vi "Open and Configure Device 4RX.vi"(0 "USRP RIO Device":T14, 5 "reference frequency source":string(combo)="Internal", 9 "Wait for GPS Lock?":bool, 11 "error in":errorcluster, 12 "rx config":T2) -> (2 "rx channels":T4={"rx config"={"channel configuration"=[], "transfer mode"=enum."Finite", "sample rate"=10000000.0, "number of samples"=8192, "start trigger"=enum."Immediate"}, "reference frequency source"="Internal", "rx.data sink"=enum."Host", "rx.enabled channels"=[], "vertical range"=[], "rx.coerced configurations"={"coerced frequencies"=[], "coerced lo frequencies"=[], "coerced levels"=[], "coerced sample rates"=[]}} {"rx.coerced configurations"."coerced sample rates" format="%#.3pS/s"; "rx.coerced configurations"."coerced levels" format="%#.3gdBm"; "rx.coerced configurations"."coerced lo frequencies" format="%#.3pHz"; "rx.coerced configurations"."coerced frequencies" format="%#.3pHz"; "rx config"."channel configuration"."channel configuration"."frequency" format="%#.3pHz"; "rx config"."channel configuration"."channel configuration"."lo frequency" format="%#.3pHz"; "rx config"."channel configuration"."channel configuration"."level" format="%#_gdBm"; "rx config"."sample rate" format="%#.3pS/s"; "vertical range" format="%#.3pVpp"}, 4 "niUsrpRio Session (out)":T5 {"Daughterboard Clock Rate" format="%#.3pHz"; "FPGA Data Clock Rate" format="%#.3pHz"; "Data Clock Rate" format="%#.3pHz"; "Characterization Data"."Frequencies [Hz]" format="%#_6p"; "EEPROM Characterization Header"."Pointer to Device Data Header" format="%x"; "EEPROM Characterization Header"."Checksum" format="%x"; "Device Data Header"."Pointer to Characterization Data" format="%x"; "Device Data Header"."Checksum" format="%x"; "EEPROM Header"."Pointer to User Header" format="%x"; "EEPROM Header"."Pointer to Factory Header" format="%x"; "EEPROM Header"."Product Code" format="%x"; "EEPROM Header"."Checksum" format="%x"}, 6 "rx.coerced configurations":T3 caption="Rx" {"coerced if2 frequencies" format="%#.3pHz"; "coerced sample rates" format="%#.3pS/s"; "coerced gain" format="%#.2f"; "coerced if1 frequencies" format="%#.3pHz"; "coerced frequencies" format="%#.3pHz"}, 15 "error out":errorcluster)   [LabVIEW 2021]
uses:
  <vilib>/userdefined/Silver/nirio_resource_slv.ctl
  <instrlib>/niUsrpRio/Config/v1/Host/Public/niUsrpRio Session.ctl
  <instrlib>/_niInstr/Register Bus/v0/Host/Public/Register Bus Session.ctl
  <instrlib>/_niInstr/Register Bus/v0/Host/Private/Session Data.ctl
  <instrlib>/niUsrpRio/Config/v1/Host/Private/DB Queue Reference.ctl
  <instrlib>/niUsrpRio/Config/v1/Host/Private/Daughterboard Data.ctl
  <instrlib>/niUsrpRio/Config/v1/Host/Private/ATR state data.ctl
  <instrlib>/niUsrpRio/Config/v1/Host/Private/Antenna Configuration.ctl
  <instrlib>/niUsrpRio/Config/v1/Host/Private/CPLD Power Mode.ctl
  <instrlib>/niUsrpRio/Config/v1/Host/Public/EEPROM Header.ctl
  <instrlib>/niUsrpRio/Config/v1/Host/Public/EEPROM Device Data Header.ctl
  <instrlib>/niUsrpRio/Config/v1/Host/Public/EEPROM Characterization Header.ctl
  <instrlib>/niUsrpRio/Config/v1/Host/Public/Characterization Data.ctl
  <instrlib>/niUsrpRio/Config/v1/Host/Public/IQ Imbalance.ctl
  Rx Channels.ctl
  Start Trigger.ctl
  <instrlib>/_niInstr/Register Bus/v0/Host/niInstr Register Bus v0 Host.lvlib
  <instrlib>/niUsrpRio/Config/v1/Host/niUsrpRio Config v1 Host.lvlib
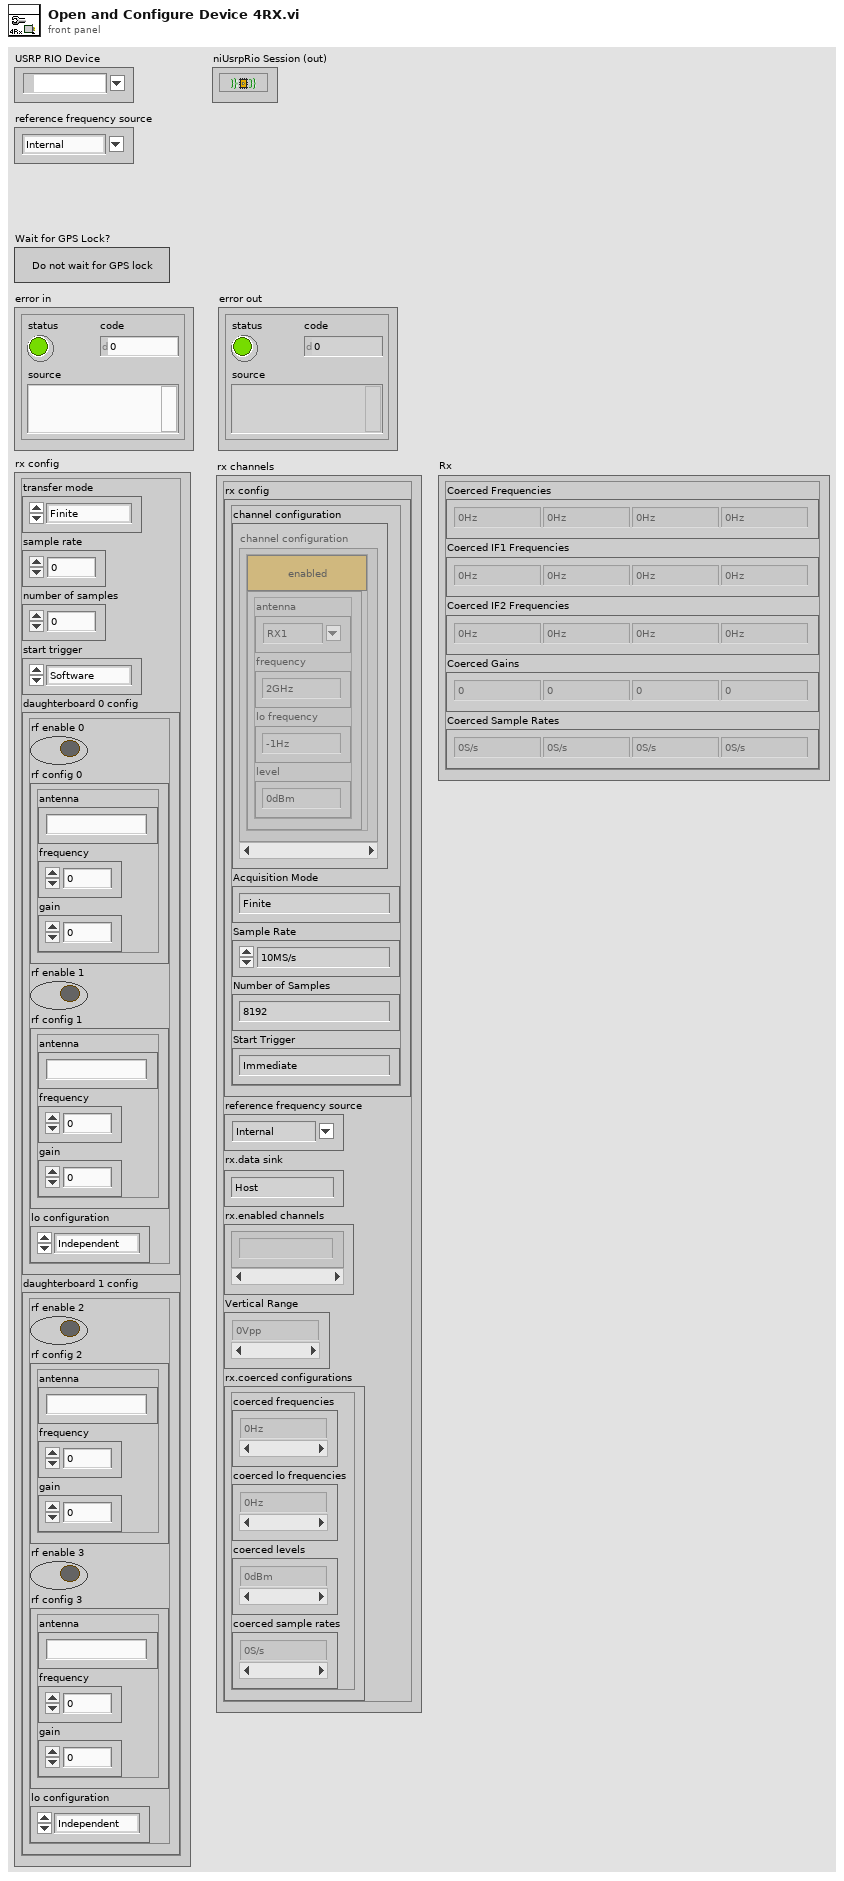
[diagram p1: front panel]
types:
  T1 = typedef "Start Trigger.ctl" = enum8{"Software", "Digital Edge", "Rx Start Trigger", "Tx Start Trigger", "Immediate", "Future Time Event"}
  T2 = cluster{"transfer mode":enum16{"Finite", "Continuous"}, "sample rate":dbl, "number of samples":u32, "start trigger":T1, "daughterboard 0 config":cluster{"rf enable 0":bool, "rf config 0":cluster{"antenna":string, "frequency":dbl, "gain":dbl}, "rf enable 1":bool, "rf config 1":cluster{"antenna":string, "frequency":dbl, "gain":dbl}, "lo configuration":enum16{"Independent", "Import", "Shared and Export", "Reimport", "Shared"}}, "daughterboard 1 config":cluster{"rf enable 2":bool, "rf config 2":cluster{"antenna":string, "frequency":dbl, "gain":dbl}, "rf enable 3":bool, "rf config 3":cluster{"antenna":string, "frequency":dbl, "gain":dbl}, "lo configuration":enum16{"Independent", "Import", "Shared and Export", "Reimport", "Shared"}}}
  T3 = cluster{"coerced frequencies":dbl[], "coerced if1 frequencies":dbl[], "coerced if2 frequencies":dbl[], "coerced gain":dbl[], "coerced sample rates":dbl[]}
  T4 = typedef "Rx Channels.ctl" = cluster{"rx config":cluster{"channel configuration":cluster{"channel enable":bool, "channel configuration":cluster{"antenna":string, "frequency":dbl, "lo frequency":dbl, "level":dbl}}[], "transfer mode":enum16{"Finite", "Continuous"}, "sample rate":dbl, "number of samples":u32, "start trigger":T1}, "reference frequency source":string, "rx.data sink":enum16{"SFP Port 0", "SFP Port 1", "Host"}, "rx.enabled channels":string[], "vertical range":dbl[], "rx.coerced configurations":cluster{"coerced frequencies":dbl[], "coerced lo frequencies":dbl[], "coerced levels":dbl[], "coerced sample rates":dbl[]}}
  T5 = typedef "niUsrpRio Config v1 Host.lvlib/niUsrpRio Session.ctl" = cluster{"FPGA Interface":refnum<k20>, "RIO Interface Number":u32, "Data Clock Rate":u32, "FPGA Data Clock Rate":u32, "Global Settings Register Bus":T6, "Radio 0 Settings Register Bus":T6, "Radio 1 Settings Register Bus":T6, "Radio Settings Bus Semaphore":T7, "DB Queues":T8[], "Characterization Data Valid?":bool, "EEPROM Header":T9, "Device Data Header":T10, "EEPROM Characterization Header":T11, "Characterization Data":T12[], "FPGA Current Version":u32, "FPGA Oldest Compatible Version":u32, "Fixed Logic Current Version":u32, "Fixed Logic Oldest Compatible Version":u32, "FPGA Radio Settings Bus Current Version":u32, "FPGA Radio Settings Bus Oldest Compatible Version":u32, "FPGA Board Config Current Version":u32, "FPGA Board Config Oldest Compatible Version":u32, "Daughterboard Clock Rate":u32, "daughterboard configuration session handles":u64[]}
  T6 = typedef "niInstr Register Bus v0 Host.lvlib/Register Bus Session.ctl" = refnum<queue>
  T7 = typedef "Semaphore RefNum" = refnum<k1>
  T8 = typedef "niUsrpRio Config v1 Host.lvlib/DB Queue Reference.ctl" = refnum<queue>
  T9 = typedef "niUsrpRio Config v1 Host.lvlib/EEPROM Header.ctl" = cluster{"Checksum":u32, "Product Code":u16, "Hardware Current Version":u16, "Hardware Oldest Compatible Version":u16, "EEPROM Map Current Version":u16, "EEPROM Map Oldest Compatible Version":u16, "User Password":string, "Pointer to Factory Header":u32, "Pointer to User Header":u32, "Recommended Interval":u16, "Number of Reserved Bytes":i32, "Number of Daughterboards":u8, "Daughterboard IDs":u16[], "Daughterboard Serial Numbers":string[]}
  T10 = typedef "niUsrpRio Config v1 Host.lvlib/EEPROM Device Data Header.ctl" = cluster{"Checksum":u32, "Number of Channels":u8, "Number of Gain Settings":u16[], "Pointer to Characterization Data":u32[], "Number of Reserved Bytes":i32, "Number of Frequencies":u16[]}
  T11 = typedef "niUsrpRio Config v1 Host.lvlib/EEPROM Characterization Header.ctl" = cluster{"Checksum":u32, "Date":timestamp, "Temperature":sgl, "Misc. Info":string, "Pointer to Device Data Header":u32, "Number of Reserved Bytes":i32}
  T12 = typedef "niUsrpRio Config v1 Host.lvlib/Characterization Data.ctl" = cluster{"Gains[dB]":dbl[], "Frequencies [Hz]":dbl[], "IQ Imbalance Table":T13[], "Measured Gains[dB]":dbl[][]}
  T13 = typedef "niUsrpRio Config v1 Host.lvlib/IQ Imbalance.ctl" = cluster{"Gain Imbalance [linear]":dbl, "Phase Imbalance [radians]":dbl, "Offset":cdb}
  T14 = typedef "nirio_resource_slv.ctl" = tag
  T15 = cluster{"channel configuration":cluster{"channel enable":bool, "channel configuration":cluster{"antenna":string, "frequency":dbl, "lo frequency":dbl, "level":dbl}}[], "transfer mode":enum16{"Finite", "Continuous"}, "sample rate":dbl, "number of samples":u32, "start trigger":T1, "tone frequency":dbl}
  T16 = cluster{"channel configuration":cluster{"channel enable":bool, "channel configuration":cluster{"antenna":string, "frequency":dbl, "lo frequency":dbl, "level":dbl}}[], "transfer mode":enum16{"Finite", "Continuous"}, "sample rate":dbl, "number of samples":u32, "start trigger":T1}
  T17 = cluster{"daughterboard 0 lo configuration":enum16{"Independent", "Import", "Shared and Export", "Reimport", "Shared"}, "daughterboard 1 lo configuration":enum16{"Independent", "Import", "Shared and Export", "Reimport", "Shared"}}
  T18 = cluster{"coerced frequencies":dbl[], "coerced lo frequencies":dbl[], "coerced levels":dbl[], "coerced sample rates":dbl[]}
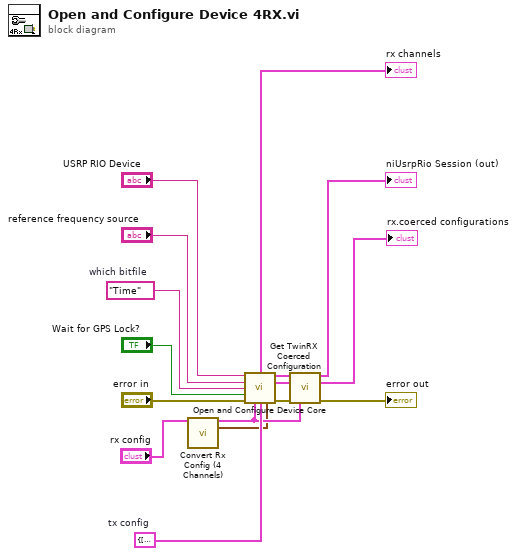
[diagram p0: block diagram]
diagram:
  w16 = "Time"  # which bitfile
  w10 = T15 {"channel configuration"=[], "transfer mode"=enum."Finite", "sample rate"=10000000.0, "number of samples"=8192, "start trigger"=enum."Immediate", "tone frequency"=100000.0}  # tx config
  n1 = call "Convert Rx Config (4 Channels).vi"("rx config"="rx config") -> ("rx config out"=w6:T16, "lo config out"=w2:T17)  [unwired: 13 in]
  n2 = call "Open and Configure Device Core.vi"("USRP RIO Device"="USRP RIO Device", "reference frequency source"="reference frequency source", "which bitfile"=w16, "wait for gps lock?"="Wait for GPS Lock?", "error in"="error in", "rx config"=w6, "tx config"=w10, "lo config"=w2) -> ("rx channels"=→"rx channels":T4, "niUsrpRio Session (out)"=w5:T5, "rx.coerced configurations"=w4:T18, "error out"=w3:errorcluster)  [unwired: 1 in, 3 out]
  n3 = call "Get TwinRX Coerced Configuration.vi"("niUsrpRio Session"=w5, "rx.coerced configurations"=w4, "error in"=w3, "rx config"=w6) -> ("niUsrpRio Session (out)"=→"niUsrpRio Session (out)":T5, "twinrx rx.coerced configurations"=→"rx.coerced configurations":T3, "error out"=→"error out":errorcluster)  [unwired: 9 in]
